vi "Features_SpecPage.vi"(10 "spec page interface":T2, 11 "metadataobj in":refnum<class "MetaDataObj.lvclass">) -> (3 "metadataobj out":refnum<class "MetaDataObj.lvclass">)   [LabVIEW 2013, in "DecideModuleFeatures.lvclass"]
uses:
  DecideModuleFeatures.lvclass
  <resource>/dialog/NewProjectWizard/Spec Page Interface.ctl
  <resource>/dialog/NewProjectWizard/MetaDataObj/MetaDataObj.lvclass
  <resource>/dialog/NewProjectWizard/MetaDataObj/MetaDataObj.lvclass/MetaDataObj.ctl
  DecideModuleFeatures.lvclass/DecideModuleFeatures.ctl
  <resource>/dialog/NewProjectWizard/MetaDataObj/Accessors/Write Project Name.vi
  <resource>/dialog/NewProjectWizard/MetaDataObj/Accessors/Write Project Root.vi
  Write component name.vi
  Write supported targets.vi
  Write supported data types.vi
  Write input_.vi
  Write output_.vi
  Write instances allowed.vi
  Write process_.vi
  <resource>/dialog/NewProjectWizard/MetaDataObj/Accessors/Write File Prefix.vi
  <vilib>/NI/Tag Bus/tag/count types.vi
  <vilib>/NI/Tag Bus/tag/index to type.vi
  <vilib>/NI/Tag Bus/tag/Data Type.ctl
  root configuration/Target Types.ctl
  root configuration/TBM configuration.lvclass
  <vilib>/NI/Tag Bus/tag/tag descriptor.lvclass
panel:
  in  "tab control":T1(tab)
  in  "Input":bool
  in  "Output":bool
  in  "Process":bool
  in  "Instances Allowed":i32=-1
  in  "Supported Targets":i32(listbox)
  in  "Available Targets":i32(listbox)
  in  "+target":bool
  in  "-target":bool
  in  "-type":bool
  in  "+type":bool
  in  "Available Data Types":i32(listbox)
  in  "Supported Data Types":i32(listbox)
  in  "module name":string
  in  "project root":path
  # "Execution Behaviors:"
  # "Produces Data (acts as an input to the system). Examples: Scan Engine, Modbus"
  # "Consumes Data (acts as an output from the system). Examples: Scan Engine, TDMS Datalogger"
  # "Processes Data (accepts data from the system and generates new data). Examples: Scaling, Alarming"
  # "Number of classes allowed in a system. Default is infinite, -1. Examples: {Scaling: -1};{Scan Engine: 1}"
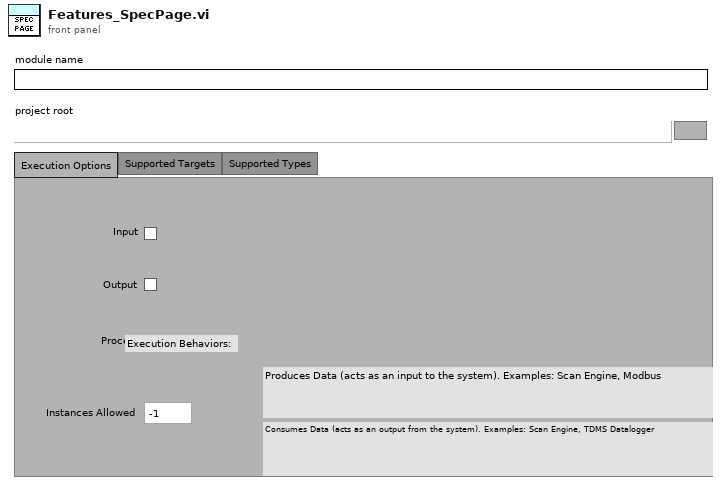
[diagram p1: front panel]
types:
  T1 = enum32{"Execution Options", "Supported Targets", "Supported Types"}
  T2 = typedef "Spec Page Interface.ctl" = cluster{"\"Tab Forward To\" Refnum":refnum<vi>, "\"Tab Backward To\" Refnum":refnum<vi>, "Errors":refnum<user-event>, "Quit":refnum<user-event>}
  T3 = typedef "TBM configuration.lvclass/Target Types.ctl" = enum16{"Windows", "Mac", "Linux", "Linux RT ARM", "VxWorks", "Pharlap", "Other", "Linux RT x64"}
  T4 = typedef "tag bus.lvlib/tag descriptor.lvclass/Data Type.ctl" = enum16{"Double", "Single", "I64", "I32", "I16", "I8", "U64", "U32", "U16", "U8", "Boolean", "String", "Array of Double", "Array of Single", "Array of I64", "Array of I32", "Array of I16", "Array of I8", "Array of U64", "Array of U32", "Array of U16", "Array of U8", "Array of Boolean", "Array of String"}
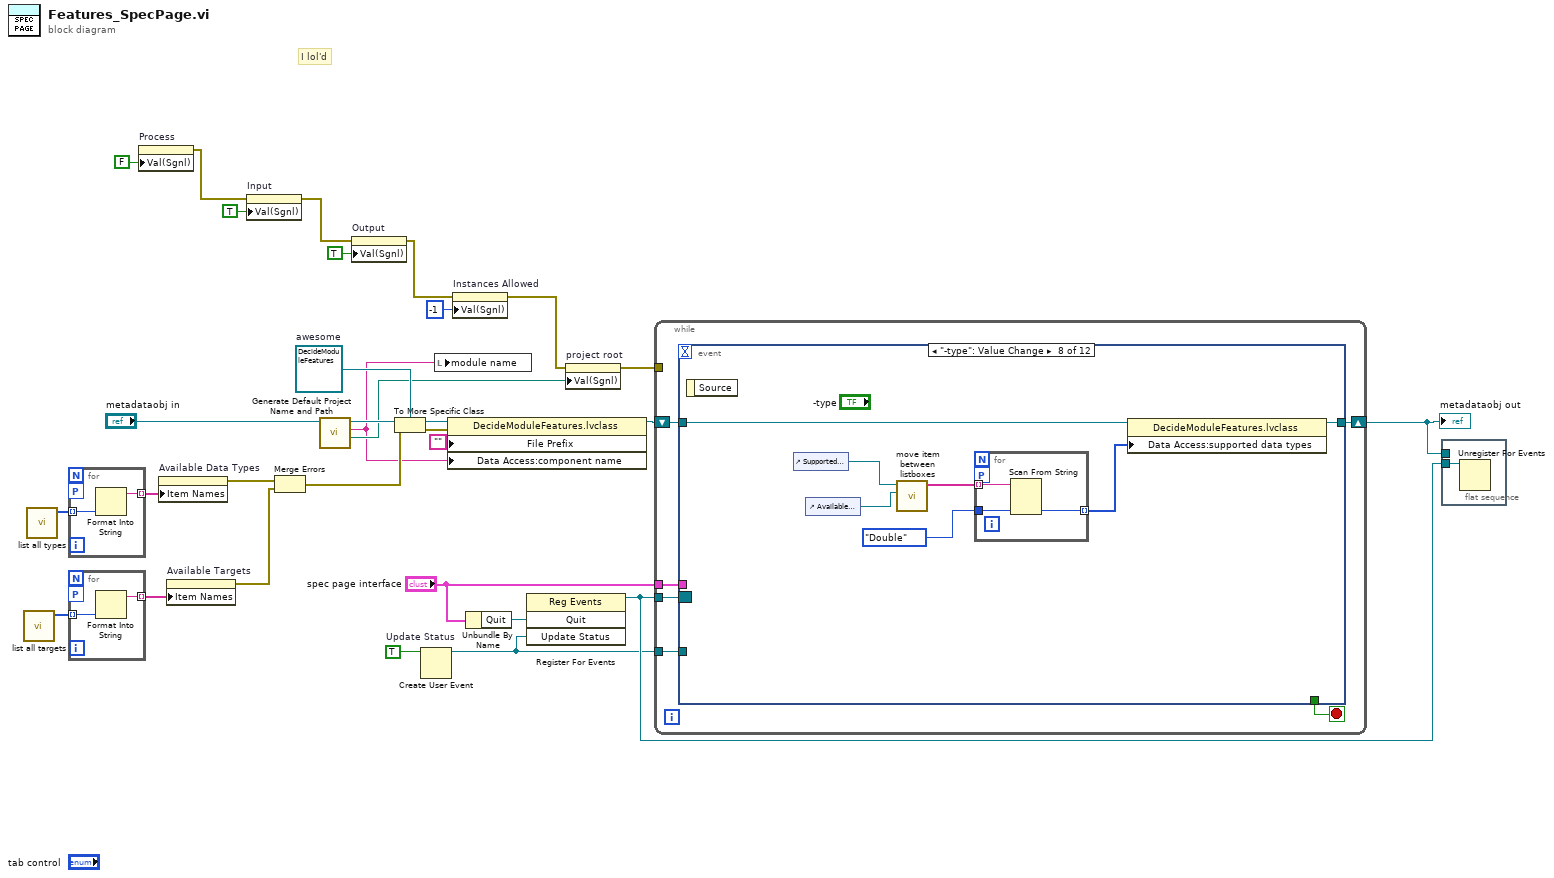
[diagram p0: block diagram]
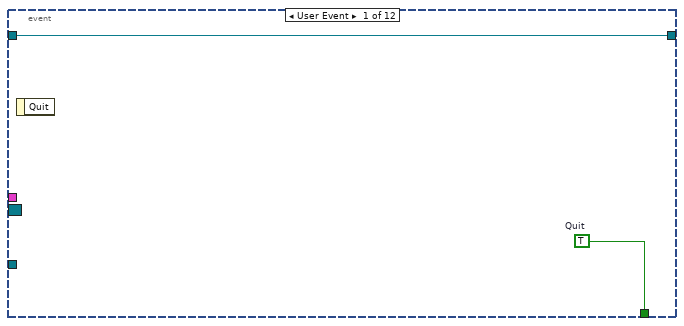
[diagram p2: hidden frame]
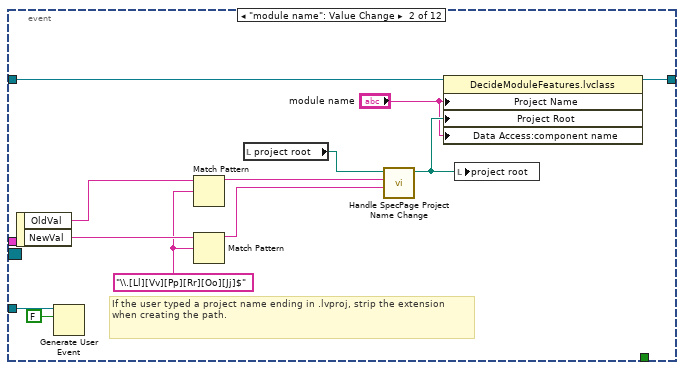
[diagram p3: hidden frame]
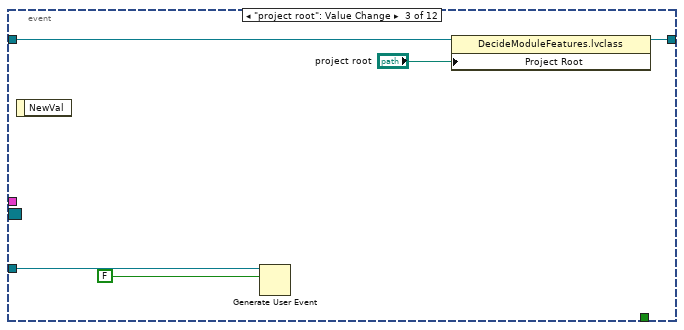
[diagram p4: hidden frame]
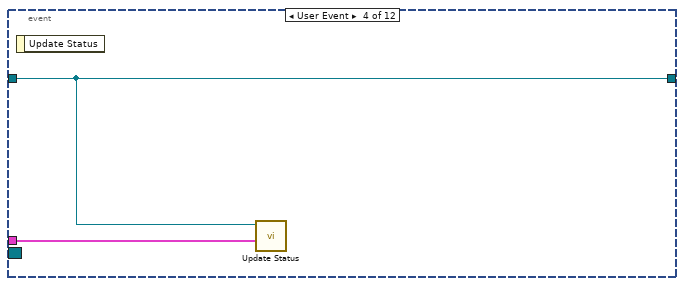
[diagram p5: hidden frame]
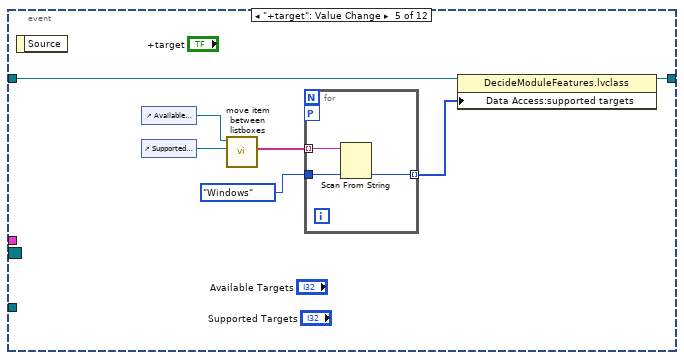
[diagram p6: hidden frame]
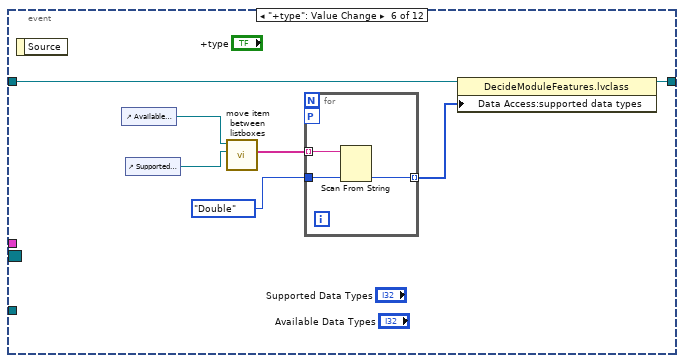
[diagram p7: hidden frame]
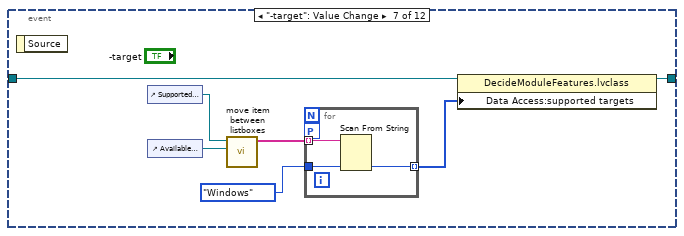
[diagram p8: hidden frame]
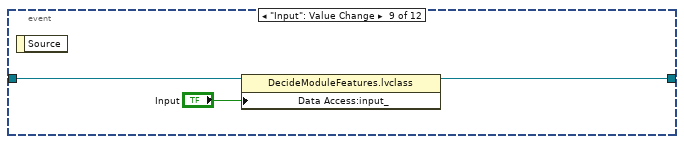
[diagram p9: hidden frame]
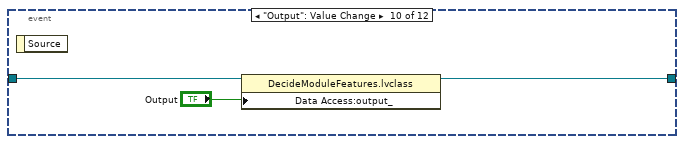
[diagram p10: hidden frame]
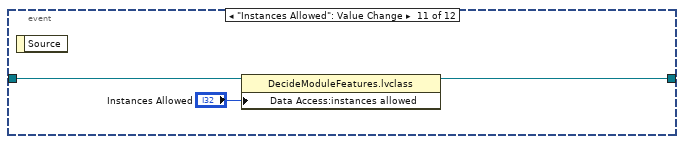
[diagram p11: hidden frame]
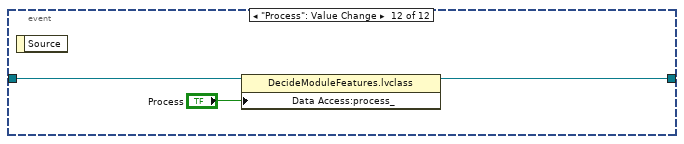
[diagram p12: hidden frame]
diagram:
  w25 = TRUE  # Update Status
  w26 = refnum<class "DecideModuleFeatures.lvclass"> refnum  # awesome
  # "I lol'd"
  n1 = call "list all targets.vi"() -> ("all targets"=w15:T3[])  [unwired: 11 in]
  n2 = call <vilib>:"list all types.vi"() -> ("all types"=w17:T4[])  [unwired: 11 in]
  n3 = for {
    tunnel: w17 -> [w33] mode=indexing
    tunnel: [w32] -> w16 mode=indexing
    workers-P: _ -> [_]
    n4 = Format Into String(w33) -> (resulting string=w32:string)  [unwired: 3 in, 1 out]
  }
  n5 = for {
    tunnel: w15 -> [w35] mode=indexing
    tunnel: [w34] -> w14 mode=indexing
    workers-P: _ -> [_]
    n6 = Format Into String(w35) -> (resulting string=w34:string)  [unwired: 3 in, 1 out]
  }
  n7 = property on="Process" class="Bool (strict)"("Val(Sgnl)"=FALSE ("Value (Signaling)")) -> (error out=w5:errorcluster)  [unwired: 2 in, 1 out]
  n8 = property on="Available Data Types" class="LstBox (strict)"("Item Names"=w16) -> (error out=w13:errorcluster)  [unwired: 2 in, 1 out]
  n9 = property on="Available Targets" class="LstBox (strict)"("Item Names"=w14) -> (error out=w12:errorcluster)  [unwired: 2 in, 1 out]
  n10 = property on="Input" class="Bool (strict)"(error in=w5, "Val(Sgnl)"=TRUE ("Value (Signaling)")) -> (error out=w6:errorcluster)  [unwired: 1 in, 1 out]
  n11 = Merge Errors(w13, w12) -> (w11:errorcluster)
  n12 = call <resource>:"Generate Default Project Name and Path.vi"("DNL_MetaDataObj in"="metadataobj in") -> ("Project Root"=w18:path, "Project Name"=w9:string, "DNL_MetaDataObj out"=w19:refnum<class "MetaDataObj.lvclass">)  [unwired: 8 in]
  n13 = property on="Output" class="Bool (strict)"(error in=w6, "Val(Sgnl)"=TRUE ("Value (Signaling)")) -> (error out=w7:errorcluster)  [unwired: 1 in, 1 out]
  n14 = To More Specific Class(target class=w26, reference=w19, error in=w11) -> (specific class reference=w28:refnum<class "DecideModuleFeatures.lvclass">, error out=w27:errorcluster)
  n15 = Create User Event(user event datatype=w25) -> (user event=w22:refnum<user-event>)  [unwired: 1 in, 1 out]
  n16 = local write "module name"(w9) -> ()
  n17 = property class="DecideModuleFeatures.lvclass"(reference=w28, error in=w27, "File Prefix"="", "Data Access:component name"=w9) -> (reference out=w24:refnum<class "DecideModuleFeatures.lvclass">)  [unwired: 1 out]
  n18 = property on="Instances Allowed" class="DigNum (strict)"(error in=w7, "Val(Sgnl)"=-1 ("Value (Signaling)")) -> (error out=w8:errorcluster)  [unwired: 1 in, 1 out]
  n19 = Unbundle By Name("spec page interface") -> ("Quit"=w31:refnum<user-event>)
  n20 = register-events(w31, w22) -> (reference out=w30:refnum<event-registration>)  [unwired: 2 in, 1 out]
  n21 = property on="project root" class="Path"(error in=w8, "Val(Sgnl)"=w18) -> (error out=w23:errorcluster)  [unwired: 1 in, 1 out]
  n22 = while {
    tunnel: "spec page interface" -> [w40]
    shift-right: [w38] -> w10
    shift-left: w24 -> [w37]
    tunnel: w30 -> [w39]
    tunnel: w23 -> [_]
    tunnel: w22 -> [w36]
    stop <- w41 stop-if-true
    n23 = event shown="[7] \"-type\": Value Change" {
      selector: w39 -> [_ _ _ _ _ _ _ _ _ _ _ _]
      dyn-events: _ -> [_ _ _ _ _ _ _ _ _ _ _ _]
      timeout: _ -> [_ _ _ _ _ _ _ _ _ _ _ _]
      tunnel: w40 -> [_ _ _ w61 _ _ _ _ _ _ _ _]
      tunnel: [w43 _ _ _ _ _ _ _ _ _ _ _] -> w41
      tunnel: [w42 w55 w59 w62 w68 w78 w88 w98 w104 w107 w110 w113] -> w38
      tunnel: w37 -> [w42 w52 w60 w62 w69 w79 w89 w99 w105 w108 w111 w114]
      tunnel: w36 -> [_ w54 w58 _ _ _ _ _ _ _ _ _]
      event User Event {
        w43 = TRUE  # Quit
        n24 = event-data() -> ()  [unwired: 1 in, 1 out]
      }
      event "module name": Value Change {
        w47 = "\\.[Ll][Vv][Pp][Rr][Oo][Jj]$" ("regular expression")
        # "If the user typed a project name ending in .lvproj, strip the extension when creating the path."
        n25 = event-data() -> ("OldVal"=w49:string, "NewVal"=w48:string)  [unwired: 1 in]
        n26 = Generate User Event(user event=w54, event data cluster=FALSE ("Update Status")) -> ()  [unwired: 2 in, 2 out]
        n27 = Match Pattern(string=w49, regular expression=w47) -> (before substring=w46:string)  [unwired: 1 in, 3 out]
        n28 = Match Pattern(string=w48, regular expression=w47) -> (before substring=w45:string)  [unwired: 1 in, 3 out]
        n29 = local read "project root"() -> (w51:path)
        n30 = call <resource>:"Handle SpecPage Project Name Change.vi"("Project Name New Value"=w45, "Project Name Old Value"=w46, "Project Root in"=w51) -> ("Project Root out"=w50:path)  [unwired: 8 in]
        n31 = property class="DecideModuleFeatures.lvclass"(reference=w52, "Project Name"="module name", "Project Root"=w50, "Data Access:component name"="module name") -> (reference out=w55:refnum<class "DecideModuleFeatures.lvclass">)  [unwired: 1 in, 1 out]
        n32 = local write "project root"(w50) -> ()
      }
      event "project root": Value Change {
        n33 = event-data() -> ()  [unwired: 1 in, 1 out]
        n34 = Generate User Event(user event=w58, event data cluster=FALSE ("Update Status")) -> ()  [unwired: 2 in, 2 out]
        n35 = property class="DecideModuleFeatures.lvclass"(reference=w60, "Project Root"="project root") -> (reference out=w59:refnum<class "DecideModuleFeatures.lvclass">)  [unwired: 1 in, 1 out]
      }
      event User Event {
        n36 = event-data() -> ()  [unwired: 1 in, 1 out]
        n37 = call "Update Status.vi"("spec page interface"=w61, "twotasksmetadataobj in"=w62) -> ()  [unwired: 10 in]
      }
      event "+target": Value Change {
        n38 = event-data() -> ()  [unwired: 1 in, 1 out]
        n39 = control-ref of="Available Targets"() -> (w67:refnum<vi>)
        n40 = control-ref of="Supported Targets"() -> (w66:refnum<vi>)
        n41 = call "move item between listboxes.vi"("target"=w66, "source"=w67) -> ("new target"=w65:string[])  [unwired: 7 in, 2 out]
        n42 = for {
          tunnel: w65 -> [w72] mode=indexing
          tunnel: Target_Types."Windows" ("Target Types") -> [w71]
          tunnel: [w70] -> w63 mode=indexing
          workers-P: _ -> [_]
          n43 = Scan From String(input string=w72, default 1=w71) -> (output 1=w70:T3)  [unwired: 3 in, 3 out]
        }
        n44 = property class="DecideModuleFeatures.lvclass"(reference=w69, "Data Access:supported targets"=w63) -> (reference out=w68:refnum<class "DecideModuleFeatures.lvclass">)  [unwired: 1 in, 1 out]
      }
      event "+type": Value Change {
        n45 = event-data() -> ()  [unwired: 1 in, 1 out]
        n46 = control-ref of="Available Data Types"() -> (w73:refnum<vi>)
        n47 = control-ref of="Supported Data Types"() -> (w75:refnum<vi>)
        n48 = call "move item between listboxes.vi"("target"=w75, "source"=w73) -> ("new target"=w77:string[])  [unwired: 7 in, 2 out]
        n49 = for {
          tunnel: w77 -> [w82] mode=indexing
          tunnel: Data_Type."Double" ("Data Type") -> [w81]
          tunnel: [w80] -> w76 mode=indexing
          workers-P: _ -> [_]
          n50 = Scan From String(input string=w82, default 1=w81) -> (output 1=w80:T4)  [unwired: 3 in, 3 out]
        }
        n51 = property class="DecideModuleFeatures.lvclass"(reference=w79, "Data Access:supported data types"=w76) -> (reference out=w78:refnum<class "DecideModuleFeatures.lvclass">)  [unwired: 1 in, 1 out]
      }
      event "-target": Value Change {
        n52 = event-data() -> ()  [unwired: 1 in, 1 out]
        n53 = control-ref of="Supported Targets"() -> (w83:refnum<vi>)
        n54 = control-ref of="Available Targets"() -> (w85:refnum<vi>)
        n55 = call "move item between listboxes.vi"("target"=w85, "source"=w83) -> ("new source"=w84:string[])  [unwired: 7 in, 2 out]
        n56 = for {
          tunnel: w84 -> [w92] mode=indexing
          tunnel: Target_Types."Windows" ("Target Types") -> [w91]
          tunnel: [w90] -> w86 mode=indexing
          workers-P: _ -> [_]
          n57 = Scan From String(input string=w92, default 1=w91) -> (output 1=w90:T3)  [unwired: 3 in, 3 out]
        }
        n58 = property class="DecideModuleFeatures.lvclass"(reference=w89, "Data Access:supported targets"=w86) -> (reference out=w88:refnum<class "DecideModuleFeatures.lvclass">)  [unwired: 1 in, 1 out]
      }
      event "-type": Value Change {
        n59 = event-data() -> ()  [unwired: 1 in, 1 out]
        n60 = control-ref of="Supported Data Types"() -> (w93:refnum<vi>)
        n61 = control-ref of="Available Data Types"() -> (w94:refnum<vi>)
        n62 = call "move item between listboxes.vi"("target"=w94, "source"=w93) -> ("new source"=w96:string[])  [unwired: 7 in, 2 out]
        n63 = for {
          tunnel: w96 -> [w102] mode=indexing
          tunnel: Data_Type."Double" ("Data Type") -> [w101]
          tunnel: [w100] -> w97 mode=indexing
          workers-P: _ -> [_]
          n64 = Scan From String(input string=w102, default 1=w101) -> (output 1=w100:T4)  [unwired: 3 in, 3 out]
        }
        n65 = property class="DecideModuleFeatures.lvclass"(reference=w99, "Data Access:supported data types"=w97) -> (reference out=w98:refnum<class "DecideModuleFeatures.lvclass">)  [unwired: 1 in, 1 out]
      }
      event "Input": Value Change {
        n66 = event-data() -> ()  [unwired: 1 in, 1 out]
        n67 = property class="DecideModuleFeatures.lvclass"(reference=w105, "Data Access:input_"="Input") -> (reference out=w104:refnum<class "DecideModuleFeatures.lvclass">)  [unwired: 1 in, 1 out]
      }
      event "Output": Value Change {
        n68 = event-data() -> ()  [unwired: 1 in, 1 out]
        n69 = property class="DecideModuleFeatures.lvclass"(reference=w108, "Data Access:output_"="Output") -> (reference out=w107:refnum<class "DecideModuleFeatures.lvclass">)  [unwired: 1 in, 1 out]
      }
      event "Instances Allowed": Value Change {
        n70 = event-data() -> ()  [unwired: 1 in, 1 out]
        n71 = property class="DecideModuleFeatures.lvclass"(reference=w111, "Data Access:instances allowed"="Instances Allowed") -> (reference out=w110:refnum<class "DecideModuleFeatures.lvclass">)  [unwired: 1 in, 1 out]
      }
      event "Process": Value Change {
        n72 = event-data() -> ()  [unwired: 1 in, 1 out]
        n73 = property class="DecideModuleFeatures.lvclass"(reference=w114, "Data Access:process_"="Process") -> (reference out=w113:refnum<class "DecideModuleFeatures.lvclass">)  [unwired: 1 in, 1 out]
      }
    }
  }
  "metadataobj out" <- w10
  n74 = flat-sequence {
    tunnel: w30 -> [w115]
    tunnel: w10 -> [_]
    frame #0 {
      n75 = Unregister For Events(event registration refnum=w115) -> ()  [unwired: 1 in, 1 out]
    }
  }
